vi "Get Shared Regs.vi"(2 "shared":refnum<class "niUSRP Rx Core v1 FPGA.lvclass">=refnum) -> ()   [LabVIEW 2023]
doc: "this VI is an accessor for Timing Information that contains the shared resource for Time-Keeping used by Alginment."
uses:
  <instrlib>/niUSRP/Reference FPGA/Rx Core/niUSRP Rx Core v1 FPGA.lvclass
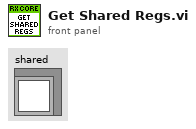
[diagram p1: front panel]
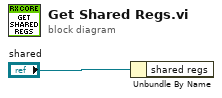
[diagram p0: block diagram]
diagram:
  n1 = Unbundle By Name("shared") -> ("shared regs"=w1)
